vi "DIAdem Error Descriptions Get.vi"(11 "internal error code":i32) -> (0 "error source":string, 1 "error code":i32, 2 "DIAdem error codes":i32[](array[numeric]), 3 "DIAdem error descriptions":string[](array[string]), 4 "type of dialog":u16(ring) items=["No dialog", "OK message", "continue or stop message"], 5 "internal code found?":bool)   [LabVIEW 2017]
doc: "This VI returns all error codes and descriptions of the LabVIEW DIAdem Connectivity VIs. You can use them with general error handler."
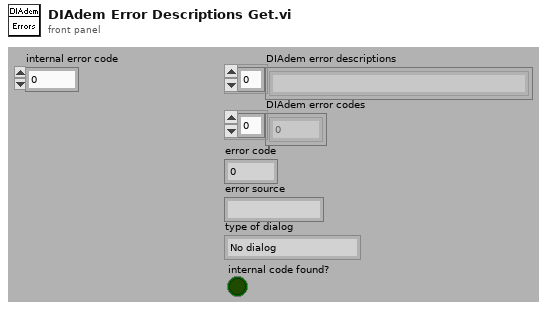
[diagram p1: front panel]
types:
  T1 = cluster{"Error code":i32, "Error description":string, "effective Error code":i32, "Error source":string, "Type of dialog":u16}[]
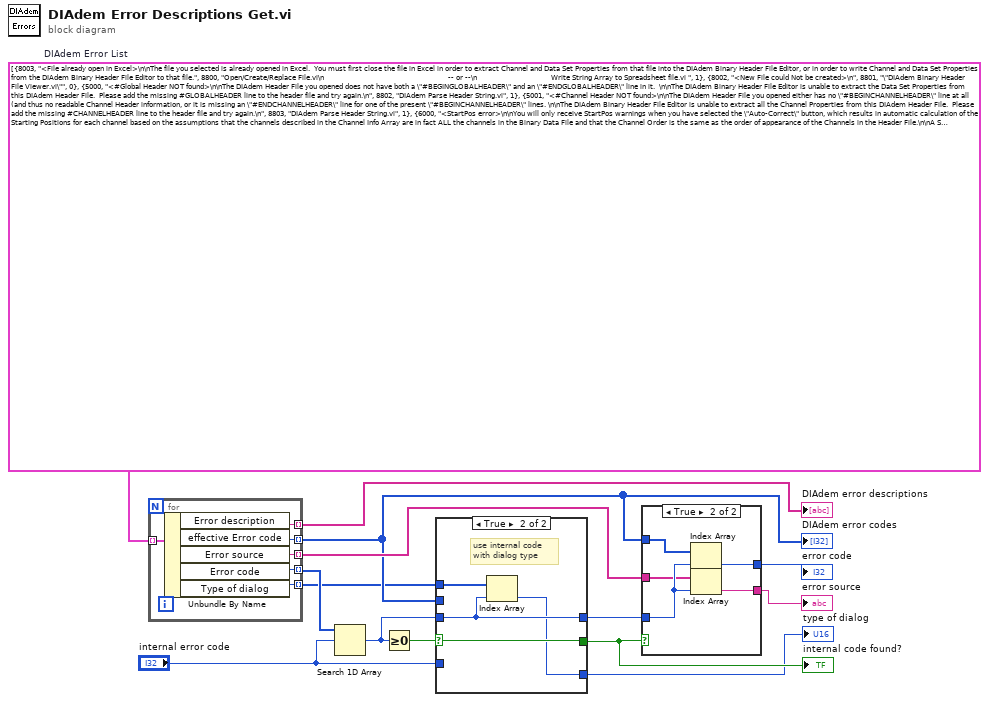
[diagram p0: block diagram]
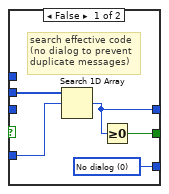
[diagram p2: hidden frame]
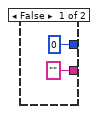
[diagram p3: hidden frame]
diagram:
  w14 = T1 [{"Error code"=8003, "Error description"="<File already open in Excel>\n\nThe file you selected is already opened in Excel.  You must first close the file in Excel in order to extract Channel and Data Set Properties from that file into the DIAdem Binary Header File Editor, or in order to write Channel and Data Set Properties from the DIAdem Binary Header File Editor to that file.", "effective Error code"=8800, "Error source"="Open/Create/Replace File.vi\n                                                              -- or --\n                                     Write String Array to Spreadsheet file.vi ", "Type of dialog"=1}, {"Error code"=8002, "Error description"="<New File could Not be created>\n", "effective Error code"=8801, "Error source"="\"DIAdem Binary Header File Viewer.vi\"", "Type of dialog"=0}, {"Error code"=5000, "Error description"="<#Global Header NOT found>\n\nThe DIAdem Header File you opened does not have both a \"#BEGINGLOBALHEADER\" and an \"#ENDGLOBALHEADER\" line in it.  \n\nThe DIAdem Binary Header File Editor is unable to extract the Data Set Properties from this DIAdem Header File.  Please add the missing #GLOBALHEADER line to the header file and try again.\n", "effective Error code"=8802, "Error source"="DIAdem Parse Header String.vi", "Type of dialog"=1}, {"Error code"=5001, "Error description"="<#Channel Header NOT found>\n\nThe DIAdem Header File you opened either has no \"#BEGINCHANNELHEADER\" line at all (and thus no readable Channel Header information, or it is missing an \"#ENDCHANNELHEADER\" line for one of the present \"#BEGINCHANNELHEADER\" lines. \n\nThe DIAdem Binary Header File Editor is unable to extract all the Channel Properties from this DIAdem Header File.  Please add the missing #CHANNELHEADER line to the header file and try again.\n", "effective Error code"=8803, "Error source"="DIAdem Parse Header String.vi", "Type of dialog"=1}, {"Error code"=6000, "Error description"="<StartPos error>\n\nYou will only receive StartPos warnings when you have selected the \"Auto-Correct\" button, which results in automatic calculation of the Starting Positions for each channel based on the assumptions that the channels described in the Channel Info Array are in fact ALL the channels in the Binary Data File and that the Channel Order is the same as the order of appearance of the Channels in the Header File.\n\nA StartPos error means that the channel generating the error was unable to interpret the number of bytes occurring before it in the binary data file (header + previous data channels) as an integral number of its data type.\n\nFor example, an R32 (SGL) channel starting after 1600 bytes of (header + prior data points) would have a starting position = 401, since from the perspective of a column of 32 bit numbers, 1600 bytes is 400 numbers'-worth, and the next position thereafter would be StartPos = 401.", "effective Error code"=8804, "Error source"="DIAdem Check--Correct Channel StartPos.vi", "Type of dialog"=1}, {"Error code"=6001, "Error description"="<BlockPos error>\n\nYou will only receive BlockPos warnings when you have selected the \"Auto-Correct\" button, which results in automatic calculation of the Starting Positions for each channel based on the assumptions that the channels described in the Channel Info Array are in fact ALL the channels in the Binary Data File and that the Channel Order is the same as the order of appearance of the Channels in the Header File.\n\nA BlockPos error means that the channel generating the error was unable to interpret the number of bytes in the binary data file between successive data points from its channel as an integral number of its data type.\n\nFor example, a SGL-SGL-DBL combination in any permutated order works fine, because each SGL column thinks the next data point belonging to it occurs 4 positions later, and the DBL column thinks the next data point belonging to it occurs 2 positions later.  Alternatively, a SGL-DBL combination is not able to be read by the DIAdem Binary Import Header, because from the DBL column's perspective, the next data point belonging to its column occurs 0.5 positions after the first, and the Import Header requires the \"Offset per Value\" to be an integer.", "effective Error code"=8805, "Error source"="DIAdem Check--Correct Channel BlockPos.vi", "Type of dialog"=1}, {"Error code"=7000, "Error description"="<Parse/Import error(s)>\n\nOne or more Channel Properties are out of range, out of order, or missing in the (*.dat) or (*.txt) DIAdem Header file you have opened.\n\nThere is a comprehensive DIAdem Header Error Report on the front panel of either \"DIAdem Read Header File.vi\" or \"DIAdem Read Header Info from Excel File.vi\" that lists all the individual Parse/Import errors and the offending text values which could not be converted.", "effective Error code"=8806, "Error source"="DIAdem Header Clusters from String Arrays.vi", "Type of dialog"=1}, {"Error code"=8004, "Error description"="Error 43 occurred at File Dialog.\n\nPossible reasons:\n\nLabVIEW:  Operation canceled by user.", "effective Error code"=8807, "Error source"="Open/Create/Replace File.vi", "Type of dialog"=0}, {"Error code"=8808, "Error description"="No DIAdem interface connection.", "effective Error code"=8808, "Error source"="DIAdem Open Reference", "Type of dialog"=2}, {"Error code"=8809, "Error description"="DIAdem is busy.", "effective Error code"=8809, "Error source"="DIAdem Report Wizard OLE Calls", "Type of dialog"=2}, {"Error code"=8810, "Error description"="DIAdem Report Wizard is not avaible.\nYou need DIAdem version 8.10 or later.", "effective Error code"=8810, "Error source"="DIAdem Report Wizard OLE Calls", "Type of dialog"=2}, {"Error code"=8811, "Error description"="DIAdem Report Wizard is not avaible.\nYou need DIAdem version 9.01 or later.", "effective Error code"=8811, "Error source"="DIAdem Report Wizard Start ", "Type of dialog"=2}, {"Error code"=8812, "Error description"="Incompatible version of DIAdem.", "effective Error code"=8812, "Error source"="DIAdem Set Value Range.vi", "Type of dialog"=2}, {"Error code"=8813, "Error description"="Setting values in DIAdem failed.", "effective Error code"=8813, "Error source"="DIAdem Set Value Range.vi", "Type of dialog"=2}, {"Error code"=8814, "Error description"="Getting values from DIAdem failed.", "effective Error code"=8814, "Error source"="DIAdem Get Value Range.vi", "Type of dialog"=2}, {"Error code"=8815, "Error description"="Setting channel length in DIAdem failed.", "effective Error code"=8815, "Error source"="Set Channel Length.vi", "Type of dialog"=1}]  # DIAdem Error List
  n1 = for {
    tunnel: w14 -> [w20] mode=indexing
    tunnel: [w19] -> w11 mode=indexing
    tunnel: [w18] -> w4 mode=indexing
    tunnel: [w17] -> w5 mode=indexing
    tunnel: [w16] -> w3 mode=indexing
    tunnel: [w15] -> w1 mode=indexing
    n2 = Unbundle By Name(w20) -> ("Error description"=w19:string, "effective Error code"=w18:i32, "Error source"=w17:string, "Error code"=w16:i32, "Type of dialog"=w15:u16)
  }
  "DIAdem error descriptions" <- w11
  "DIAdem error codes" <- w4
  n3 = Search 1D Array(1D array=w3, element="internal error code") -> (index of element=w9:i32)  [unwired: 1 in]
  n4 = Greater Or Equal To 0?(x=w9) -> (x >= 0?=w10:bool)
  n5 = case shown="True" w10 {
    selector: w10 -> [_ w29]
    tunnel: w9 -> [_ w27]
    tunnel: [w22 w27] -> w8
    tunnel: w4 -> [w25 _]
    tunnel: "internal error code" -> [w24 _]
    tunnel: [w23 w29] -> w6
    tunnel: w1 -> [_ w28]
    tunnel: [w21 w26] -> w2
    frame False {
      w21 = u16 0 items=["No dialog", "OK message", "continue or stop message"] ("Type of dialog")
      # "search effective code (no dialog to prevent duplicate messages)"
      n6 = Search 1D Array(1D array=w25, element=w24) -> (index of element=w22:i32)  [unwired: 1 in]
      n7 = Greater Or Equal To 0?(x=w22) -> (x >= 0?=w23:bool)
    }
    frame True {
      # "use internal code with dialog type"
      n8 = Index Array(array=w28, index=w27) -> (element=w26:u16)
    }
  }
  "internal code found?" <- w6
  "type of dialog" <- w2
  n9 = case shown="True" w6 {
    tunnel: w8 -> [_ w36]
    tunnel: w4 -> [_ w32]
    tunnel: w5 -> [_ w35]
    tunnel: [0 ("effective Error code") w34] -> w13
    tunnel: ["" ("Error source") w33] -> w12
    frame False {
    }
    frame True {
      n10 = Index Array(array=w32, index=w36) -> (element=w34:i32)
      n11 = Index Array(array=w35, index=w36) -> (element=w33:string)
    }
  }
  "error code" <- w13
  "error source" <- w12
